vi "Null Broadcast Events--constant.vi"() -> (3 "Acquisition Broadcast Events":T1)   [LabVIEW 2016, in "Acquisition.lvlib"]
doc: "Returns the broadcast events cluster with null references for defining the event types in a Register For Events function.\n_____\nBased on DQMH Project Template 6.1.0.94."
uses:
  Acquisition.lvlib
  Broadcast Events--cluster.ctl
  Did Init Argument--cluster.ctl
  Status Updated Argument--cluster.ctl
  Error Reported Argument--cluster.ctl
  Stop Argument--cluster.ctl
  Get Module Execution Status Argument--cluster.ctl
  Acquisition Started Argument--cluster.ctl
  Acquisition Stopped Argument--cluster.ctl
  Data Updated Argument--cluster.ctl
  Device Calibrated Argument--cluster.ctl
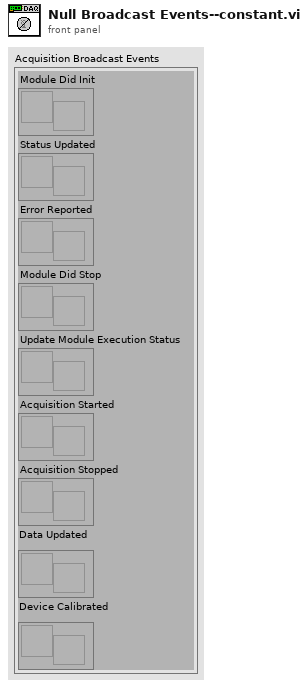
[diagram p1: front panel]
types:
  T1 = typedef "Acquisition.lvlib/Broadcast Events--cluster.ctl" = cluster{"Module Did Init":refnum<user-event>, "Status Updated":refnum<user-event>, "Error Reported":refnum<user-event>, "Module Did Stop":refnum<user-event>, "Update Module Execution Status":refnum<user-event>, "Acquisition Started":refnum<user-event>, "Acquisition Stopped":refnum<user-event>, "Data Updated":refnum<user-event>, "Device Calibrated":refnum<user-event>}
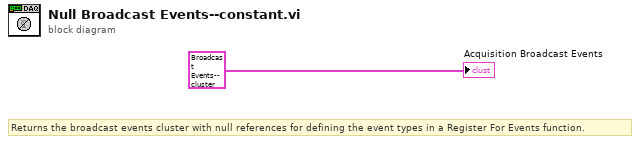
[diagram p0: block diagram]
diagram:
  # "Returns the broadcast events cluster with null references for defining the event types in a Register For Events function."
  "Acquisition Broadcast Events" <- T1 {"Module Did Init"=refnum, "Status Updated"=refnum, "Error Reported"=refnum, "Module Did Stop"=refnum, "Update Module Execution Status"=refnum, "Acquisition Started"=refnum, "Acquisition Stopped"=refnum, "Data Updated"=refnum, "Device Calibrated"=refnum} ("Broadcast Events")
